vi "AI 9213-Thremocouple Test.vi"() -> ()   [LabVIEW 2021]
uses:
  <vilib>/DAQmx/read.llb/DAQmx Read (Analog 1D Wfm NChan NSamp).vi
  <vilib>/DAQmx/create/channels.llb/DAQmx Create Channel (AI-Temperature-Thermocouple).vi
  <vilib>/DAQmx/configure/timing.llb/DAQmx Timing (Sample Clock).vi
  <vilib>/DAQmx/miscellaneous.llb/DAQmx Fill In Error Info.vi
  <resource>/objmgr/daqmx.rc
panel:
  out "Daq mx Read Rate":dbl
  out "x-y":u32
  in  "error in (no error)":errorcluster
  out "SampClk.MaxRate":dbl
  out "Configuring Channel":tag[](array[tag])
  out "ms  to Wait":u32
  in  "units":i32(ring)=10143 items=["Deg C"=10143, "Deg F"=10144, "Kelvins"=10325, "Deg R"=10145, "From Custom Scale"=10065]
  in  "thermocouple type":i32(ring)=10072 items=["J"=10072, "K"=10073, "N"=10077, "R"=10082, "S"=10085, "T"=10086, "B"=10047, "E"=10055]
  in  "rate":dbl=1000.0 format="%0.2f"
  in  "samples per channel":i32=1000
  in  "sample mode":i32(ring)=10178 items=["Finite Samples"=10178, "Continuous Samples"=10123, "Hardware Timed Single Point"=12522]
  in  "minimum value":dbl=-5.0 format="%#_13g"
  in  "maximum value":dbl=5.0 format="%#_13g"
  in  "Stop":bool
  out "data":waveform(dbl)[](array[waveform])
  out "Waveform Chart":waveform(dbl)[](graph)
  out "Waveform Graph":waveform(dbl)[](graph)
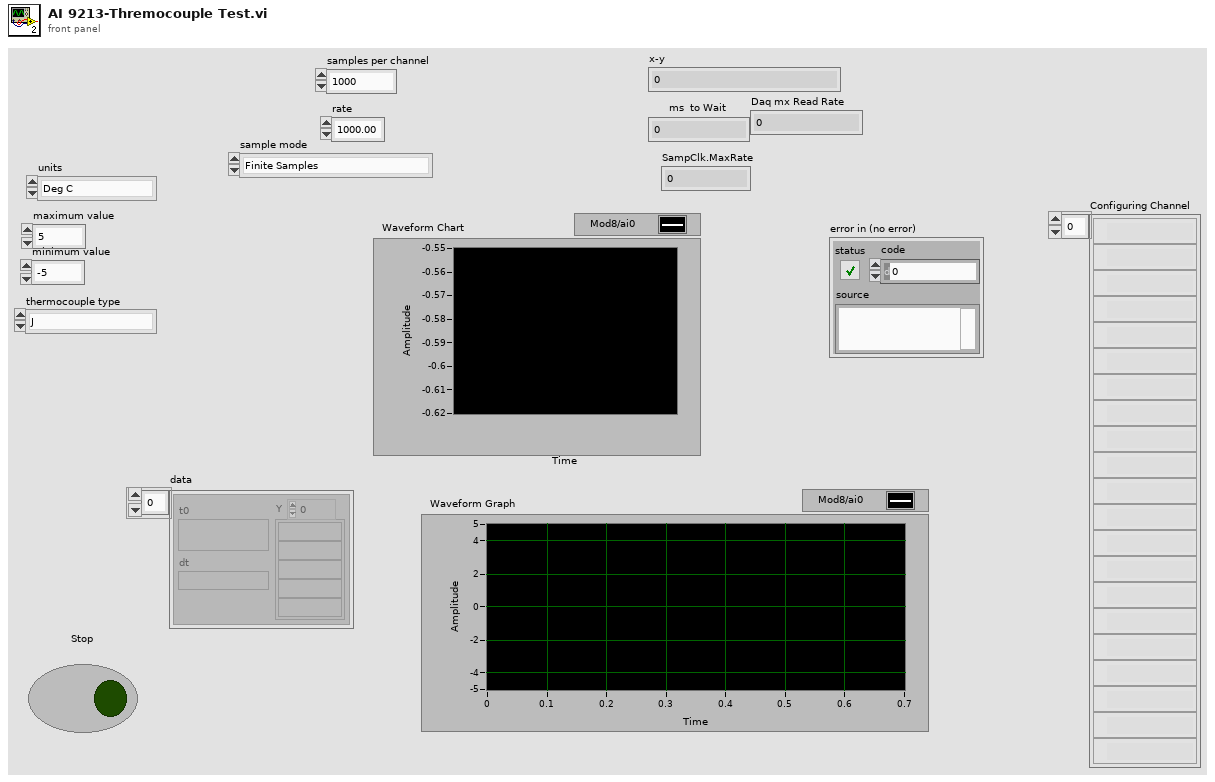
[diagram p1: front panel]
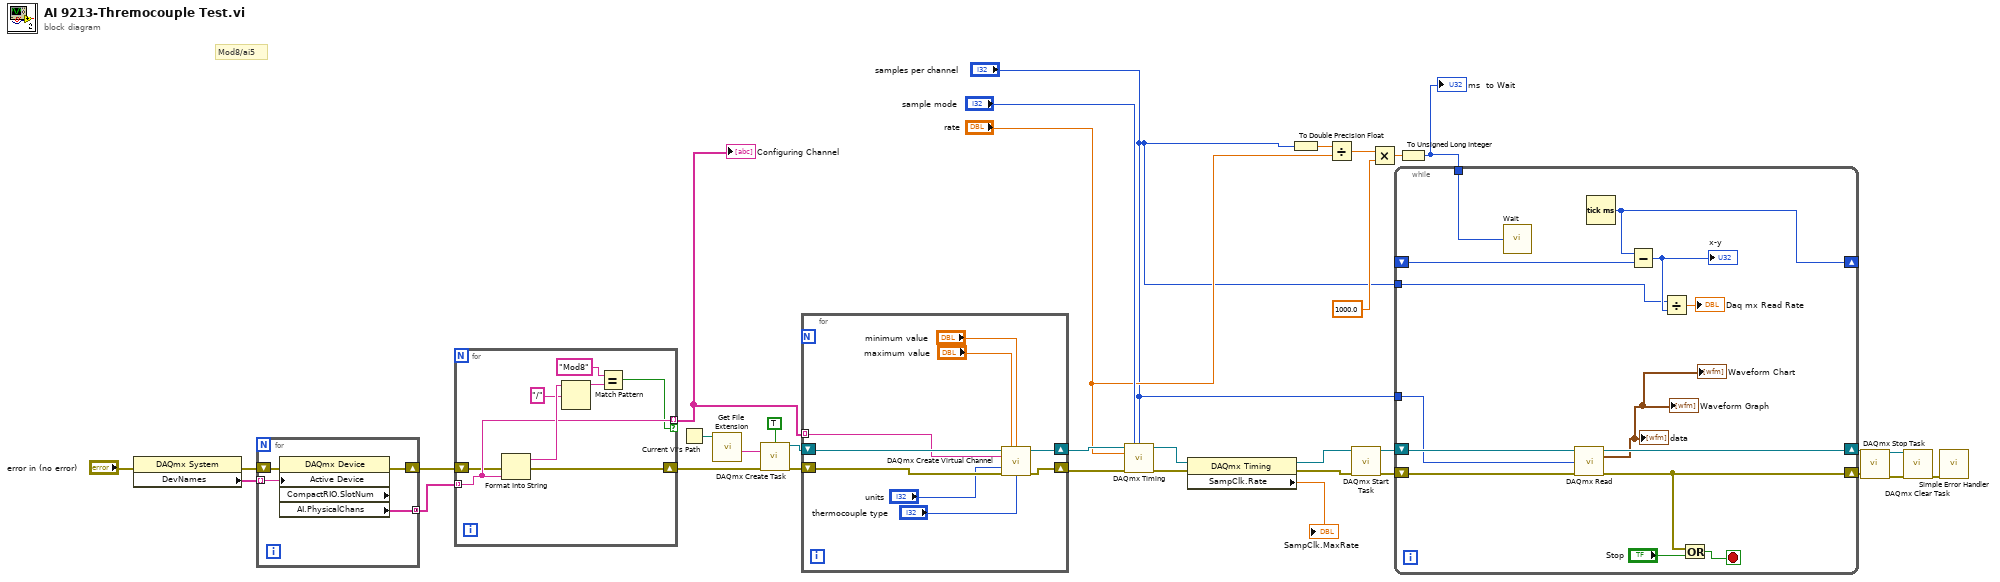
[diagram p0: block diagram]
diagram:
  # "Mod8/ai5"
  n1 = property class="DAQmx System"(error in="error in (no error)") -> (error out=w30:errorcluster, "DevNames"=w34:tag[])  [unwired: 1 in, 1 out]
  n2 = for {
    tunnel: w34 -> [w38] mode=indexing
    shift-right: [w37] -> w5
    shift-left: w30 -> [w36]
    tunnel: [w35] -> w13 mode=concatenating
    n3 = property class="DAQmx Device" props=["Active Device", "CompactRIO.SlotNum", "AI.PhysicalChans"](error in=w36, "Active Device"=w38) -> (error out=w37:errorcluster, "AI.PhysicalChans"=w35:tag[])  [unwired: 1 in, 2 out]
  }
  n4 = for {
    tunnel: w13 -> [w42] mode=indexing
    tunnel: [w42] -> w12 mode=indexing if=w41
    shift-right: [w39] -> w4
    shift-left: w5 -> [w40]
    n5 = Format Into String(error in=w40, w42) -> (resulting string=w46:string, error out=w39:errorcluster)  [unwired: 2 in]
    n6 = Match Pattern(string=w46, regular expression="/") -> (before substring=w44:string)  [unwired: 1 in, 3 out]
    n7 = Equal?(x="Mod8" ("regular expression"), y=w44) -> (x = y?=w41:bool)
  }
  "Configuring Channel" <- w12
  n8 = Current VI's Path() -> (path=w3:path)
  n9 = call <vilib>:"Get File Extension.vi"("file"=w3) -> ("filename without extension"=w2:string)  [unwired: 6 in, 4 out]
  n10 = call <vilib>:"DAQmx Create Task.vi"("new task name"=w2, "auto cleanup"=TRUE, "error in"=w4) -> ("task out"=w31:refnum<k21>, "error out"=w32:errorcluster)  [unwired: 11 in]
  n11 = for {
    shift-right: [w51] -> w22
    shift-left: w32 -> [w55]
    shift-right: [w50] -> w21
    shift-left: w31 -> [w54]
    tunnel: w12 -> [w47] mode=indexing
    n12 = call-poly <vilib>:"DAQmx Create Virtual Channel.vi"("task in"=w54, "maximum value"="maximum value", "minimum value"="minimum value", "physical channels"=w47, "units"="units", "error in"=w55, "thermocouple type"="thermocouple type") -> ("task out"=w50:refnum<k21>, "error out"=w51:errorcluster)  [unwired: 7 in]
  }
  n13 = call-poly <vilib>:"DAQmx Timing.vi"("task/channels in"=w21, "sample mode"="sample mode", "samples per channel"="samples per channel", "rate"="rate", "error in"=w22) -> ("task out"=w11:refnum<k21>, "error out"=w9:errorcluster)  [unwired: 9 in]
  n14 = property class="DAQmx Timing"(reference=w11, error in=w9) -> (reference out=w7:refnum<k21>, error out=w8:errorcluster, "SampClk.Rate"=→"SampClk.MaxRate":dbl)
  n15 = To Double Precision Float(number="samples per channel") -> (double precision float=w16:dbl)
  n16 = Divide(x=w16, y="rate") -> (x/y=w18:dbl)
  n17 = call <vilib>:"DAQmx Start Task.vi"("task/channels in"=w7, "error in"=w8) -> ("task out"=w29:refnum<k21>, "error out"=w28:errorcluster)  [unwired: 12 in]
  n18 = Multiply(x=w18, y=1000.0) -> (x*y=w17:dbl)
  n19 = To Unsigned Long Integer(number=w17) -> (unsigned 32bit integer=w14:u32)
  "ms  to Wait" <- w14
  n20 = while {
    shift-right: [w64] -> w24
    shift-left: w29 -> [w67]
    shift-right: [w65] -> w27
    shift-left: w28 -> [w66]
    tunnel: "samples per channel" -> [w63]
    tunnel: w14 -> [w61]
    shift-right: [w59] -> _
    shift-left: _ -> [w60]
    tunnel: "samples per channel" -> [w56]
    stop <- w68 stop-if-true
    n21 = call "Wait"("Count(mSec)"=w61) -> ()  [unwired: 1 out]
    n22 = call-poly <vilib>:"DAQmx Read.vi"("task/channels in"=w67, "number of samples per channel"=w63, "error in"=w66) -> ("task out"=w64:refnum<k21>, "data"=→"data" →"Waveform Chart" →"Waveform Graph":waveform(dbl)[], "error out"=w65:errorcluster)  [unwired: 10 in]
    n23 = Tick Count (ms)() -> (millisecond timer value=w59:u32)
    n24 = Subtract(x=w59, y=w60) -> (x-y=w57:u32)
    "x-y" <- w57
    n25 = Divide(x=w56, y=w57) -> (x/y=→"Daq mx Read Rate":dbl)
    n26 = Or(x=w65, y="Stop") -> (x .or. y?=w68:bool)
  }
  n27 = call <vilib>:"DAQmx Stop Task.vi"("task/channels in"=w24, "error in"=w27) -> ("task out"=w23:refnum<k21>, "error out"=w26:errorcluster)  [unwired: 12 in]
  n28 = call <vilib>:"DAQmx Clear Task.vi"("task in"=w23, "error in"=w26) -> ("error out"=w25:errorcluster)  [unwired: 13 in]
  n29 = call <vilib>:"Simple Error Handler.vi"("error in (no error)"=w25) -> ()  [unwired: 4 in, 5 out]
